vi "Coord window-Set menu tick marks.vi"(8 "error in (no error)":errorcluster, 11 "Menu in":refnum<k9>) -> (0 "error out":errorcluster, 3 "Menu out":refnum<k9>)   [LabVIEW 2017]
uses:
  Typedefs/Movement mode.ctl
  Position control window/Globals/Pos ctrl window globals.vi
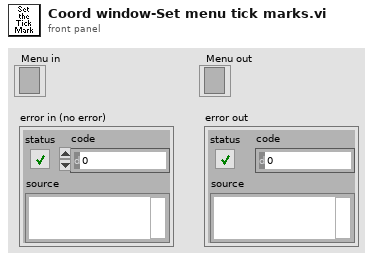
[diagram p1: front panel]
types:
  T1 = typedef "Movement mode.ctl" = enum16{"Move the frame", "Move the feature"}
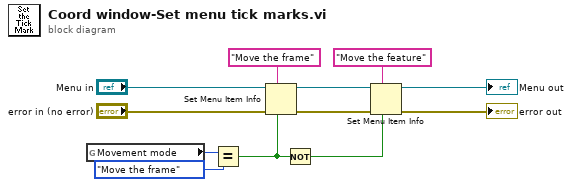
[diagram p0: block diagram]
diagram:
  n1 = global read "Pos ctrl window globals.vi" "Movement mode"() -> (w1:T1)
  n2 = Equal?(x=w1, y=Movement_mode."Move the frame") -> (x = y?=w11:bool)
  n3 = Set Menu Item Info(6:w11, 7:"Move the frame" ("item tag"), 8:"error in (no error)", 11:"Menu in") -> (0:→"error out":errorcluster, 3:w8:refnum<k9>)  [unwired: 3 in]
  n4 = Not(x=w11) -> (.not. x?=w10:bool)
  n5 = Set Menu Item Info(6:w10, 7:"Move the feature" ("item tag"), 11:w8) -> (3:→"Menu out":refnum<k9>)  [unwired: 4 in, 1 out]
